vi "002_DataMonitor.vi"(11 "Queue Ref":T1={"UI"=refnum, "Message"=refnum, "Data"=refnum, "Caller"=refnum, "Name"="000 Common", "Data Path"=path "", "Class Path"=path "", "SubPanel"=refnum, "Project Name"="", "MNT"="", "Title"="", "Data Source"=refnum, "Queue List"={}, "VI"=refnum, "UE"=refnum}) -> ()   [LabVIEW 2020]
doc: "1212"
uses:
  Alin/QMH/000 Module Data Type.ctl
  Alin/QMH/Queue Message.ctl
  0007 Controls/Data Module.ctl
  0007 Controls/Data Modules.ctl
  0007 Controls/Data Element Single.ctl
  <vilib>/Utility/miscctls.llb/LVPointTypeDef.ctl
panel:
  out "QN":i32
  in  "Modules":T2={"Module01"={"Names"={"Module Name"="", "Set Value"="", "Real Value"="", "FB Value"="", "Unit"="", "Identifier"="", "IdentifierW"="写入标识符", "Decimal"="位数", "AS"=FALSE, "AR"=FALSE, "Con"=FALSE}, "Data"=[], "Digit"=0.0}, "Module02"={"Names"={"Module Name"="", "Set Value"="", "Real Value"="", "FB Value"="", "Unit"="", "Identifier"="", "IdentifierW"="写入标识符", "Decimal"="位数", "AS"=FALSE, "AR"=FALSE, "Con"=FALSE}, "Data"=[], "Digit"=0.0}, "Module03"={"Names"={"Module Name"="", "Set Value"="", "Real Value"="", "FB Value"="", "Unit"="", "Identifier"="", "IdentifierW"="写入标识符", "Decimal"="位数", "AS"=FALSE, "AR"=FALSE, "Con"=FALSE}, "Data"=[], "Digit"=0.0}, "Module04"={"Names"={"Module Name"="", "Set Value"="", "Real Value"="", "FB Value"="", "Unit"="", "Identifier"="", "IdentifierW"="写入标识符", "Decimal"="位数", "AS"=FALSE, "AR"=FALSE, "Con"=FALSE}, "Data"=[], "Digit"=0.0}, "Module05"={"Names"={"Module Name"="", "Set Value"="", "Real Value"="", "FB Value"="", "Unit"="", "Identifier"="", "IdentifierW"="写入标识符", "Decimal"="位数", "AS"=FALSE, "AR"=FALSE, "Con"=FALSE}, "Data"=[], "Digit"=0.0}, "Module06"={"Names"={"Module Name"="", "Set Value"="", "Real Value"="", "FB Value"="", "Unit"="", "Identifier"="", "IdentifierW"="写入标识符", "Decimal"="位数", "AS"=FALSE, "AR"=FALSE, "Con"=FALSE}, "Data"=[], "Digit"=0.0}, "Module07"={"Names"={"Module Name"="", "Set Value"="", "Real Value"="", "FB Value"="", "Unit"="", "Identifier"="", "IdentifierW"="写入标识符", "Decimal"="位数", "AS"=FALSE, "AR"=FALSE, "Con"=FALSE}, "Data"=[], "Digit"=0.0}, "Module08"={"Names"={"Module Name"="", "Set Value"="", "Real Value"="", "FB Value"="", "Unit"="", "Identifier"="", "IdentifierW"="写入标识符", "Decimal"="位数", "AS"=FALSE, "AR"=FALSE, "Con"=FALSE}, "Data"=[], "Digit"=0.0}, "Module09"={"Names"={"Module Name"="", "Set Value"="", "Real Value"="", "FB Value"="", "Unit"="", "Identifier"="", "IdentifierW"="写入标识符", "Decimal"="位数", "AS"=FALSE, "AR"=FALSE, "Con"=FALSE}, "Data"=[], "Digit"=0.0}, "Module10"={"Names"={"Module Name"="", "Set Value"="", "Real Value"="", "FB Value"="", "Unit"="", "Identifier"="", "IdentifierW"="写入标识符", "Decimal"="位数", "AS"=FALSE, "AR"=FALSE, "Con"=FALSE}, "Data"=[], "Digit"=0.0}, "Module11"={"Names"={"Module Name"="", "Set Value"="", "Real Value"="", "FB Value"="", "Unit"="", "Identifier"="", "IdentifierW"="写入标识符", "Decimal"="位数", "AS"=FALSE, "AR"=FALSE, "Con"=FALSE}, "Data"=[], "Digit"=0.0}}
  in  "Module Add":bool
  in  "Panel Show":bool
  in  "Panel Refresh":bool
  in  "Show Config":bool
  out "Warning":string
  in  "Horizontal scroll bar":bool caption="H"
  in  "Vertical scroll bar":bool caption="V"
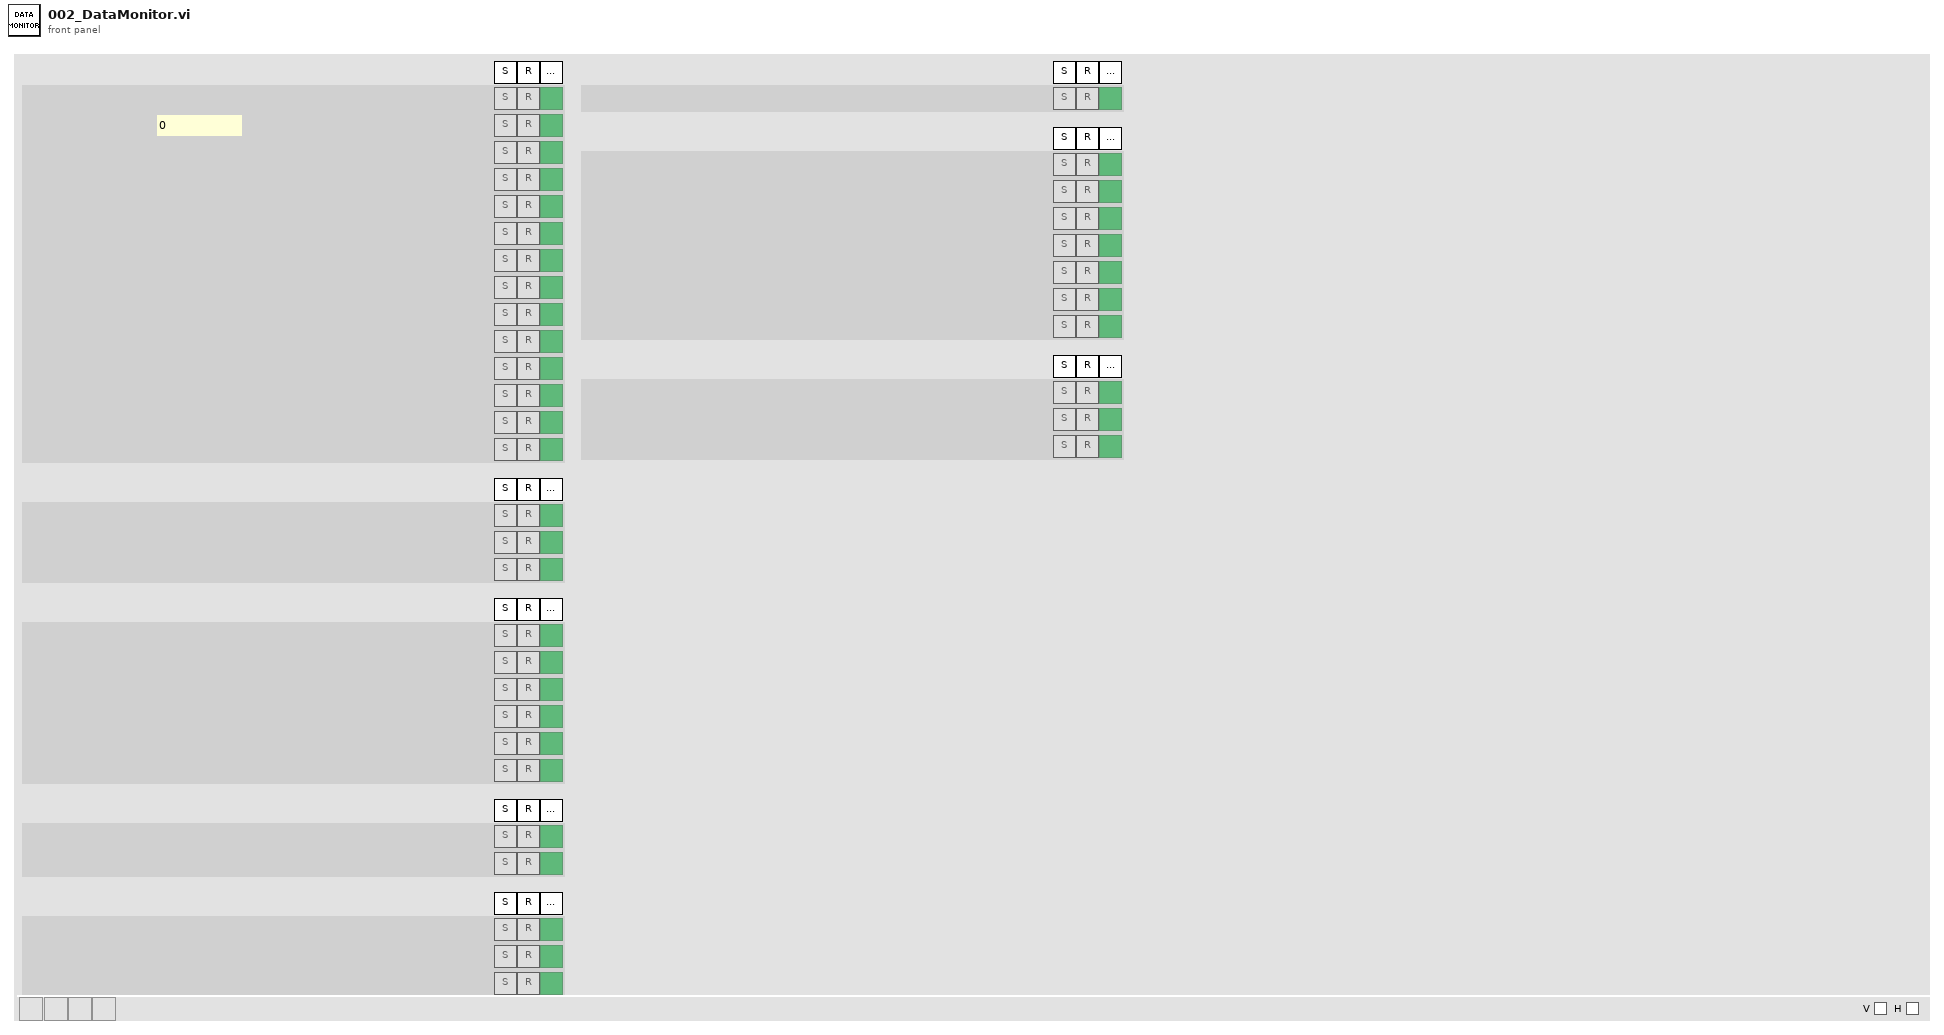
[diagram p1: front panel]
types:
  T1 = typedef "000 Module Data Type.ctl" = cluster{"UI":refnum<queue>, "Message":refnum<queue>, "Data":refnum<queue>, "Caller":refnum<queue>, "Name":string, "Data Path":path, "Class Path":path, "SubPanel":refnum<vi>, "Project Name":string, "MNT":string, "Title":string, "Data Source":refnum<queue>, "Queue List":map{string, refnum<queue>}, "VI":refnum<vi>, "UE":refnum<user-event>}
  T2 = typedef "Data Module.ctl" = cluster{"Module01":T3, "Module02":T3, "Module03":T3, "Module04":T3, "Module05":T3, "Module06":T3, "Module07":T3, "Module08":T3, "Module09":T3, "Module10":T3, "Module11":T3}
  T3 = typedef "Data Modules.ctl" = cluster{"Names":cluster{"Module Name":string, "Set Value":string, "Real Value":string, "FB Value":string, "Unit":string, "Identifier":string, "IdentifierW":string, "Decimal":string, "AS":bool, "AR":bool, "Con":bool}, "Data":T4[], "Digit":dbl}
  T4 = typedef "Data Element Single.ctl" = cluster{"Name":string, "Set Value":string, "Real Value":string, "FB Value":string, "Unit":string, "Identifier":string, "Write Name":string, "Decimal":u16, "AS":bool, "AR":bool, "ALM":bool, "Up":bool, "Down":bool}
  T5 = cluster{"Queue Ref":T1, "Modules":T2, "Count Time(ms)":u32, "Delay Time(ms)":u32, "Next":string, "WarningID":string[]}
  T6 = cluster{"Modules[0]":T3, "Modules[1]":T3, "Modules[2]":T3, "Modules[3]":T3, "Modules[4]":T3, "Modules[5]":T3, "Modules[6]":T3, "Modules[7]":T3, "Modules[8]":T3, "Modules[9]":T3, "Modules[10]":T3}
  T7 = typedef "SDQ Data Type.ctl" = cluster{"CAN Length":string, "CAN Name":string, "CAN ID":string, "CAN Type":string, "Test Item":string, "Byte Order":string, "Instruction":string, "Control Type":string, "Group":string, "Offset":dbl, "Coefficient":dbl, "Write Enable":bool, "Lable Type":string, "Key?":string, "Set Value":string, "Upper":dbl, "Lower":dbl, "Unit":string, "Formula":string, "Test Item Type":string, "Length":i32, "Address":string, "Name":string, "Identifier":string, "Data Type":string, "Enumerate?":string, "Enumerate List":string, "Data":string, "Source":string}
  T8 = cluster{"[0]":T3, "[1]":T3, "[2]":T3, "[3]":T3, "[4]":T3, "[5]":T3, "[6]":T3, "[7]":T3, "[8]":T3, "[9]":T3, "[10]":T3}
  T9 = typedef "eventvkey.ctl" = enum16{"ASCII", "Enter", "Return", "Shift", "Ctrl", "Alt", "Cmd", "Opt", "Caps", "NumLock", "Clear", "Break", "Up", "Down", "Left", "Right", "Insert", "Delete", "Home", "End", "PageUp", "PageDown", "Escape", "Help", "Pause", "ScrollLock", "F1", "F2", "F3", "F4", "F5", "F6", "F7", "F8", "F9", "F10", "F11", "F12", "F13", "F14", "F15", "F16", "F17", "F18", "F19", "F20", "F21", "F22", "F23", "F24", "Play", "VolumeUp", "VolumeDown", "Mute", "Two Byte Char"}
  T10 = cluster{"Shift":bool, "Ctrl":bool, "Alt":bool, "Cmd":bool, "Opt":bool}
  T11 = typedef "LVPoint32TypeDef.ctl" = cluster{"Horizontal":i32, "Vertical":i32}
  T12 = cluster{"Queue List":map{string, refnum<queue>}, "SubPanel":refnum<vi>, "Active Panel":string, "Queue Ref":T1, "Project Name":string, "ModulesRef":refnum<vi>, "Vertical scroll bar":bool, "Horizontal scroll bar":bool}
  T13 = typedef "LVPointTypeDef.ctl" = cluster{"Horizontal":i16, "Vertical":i16}
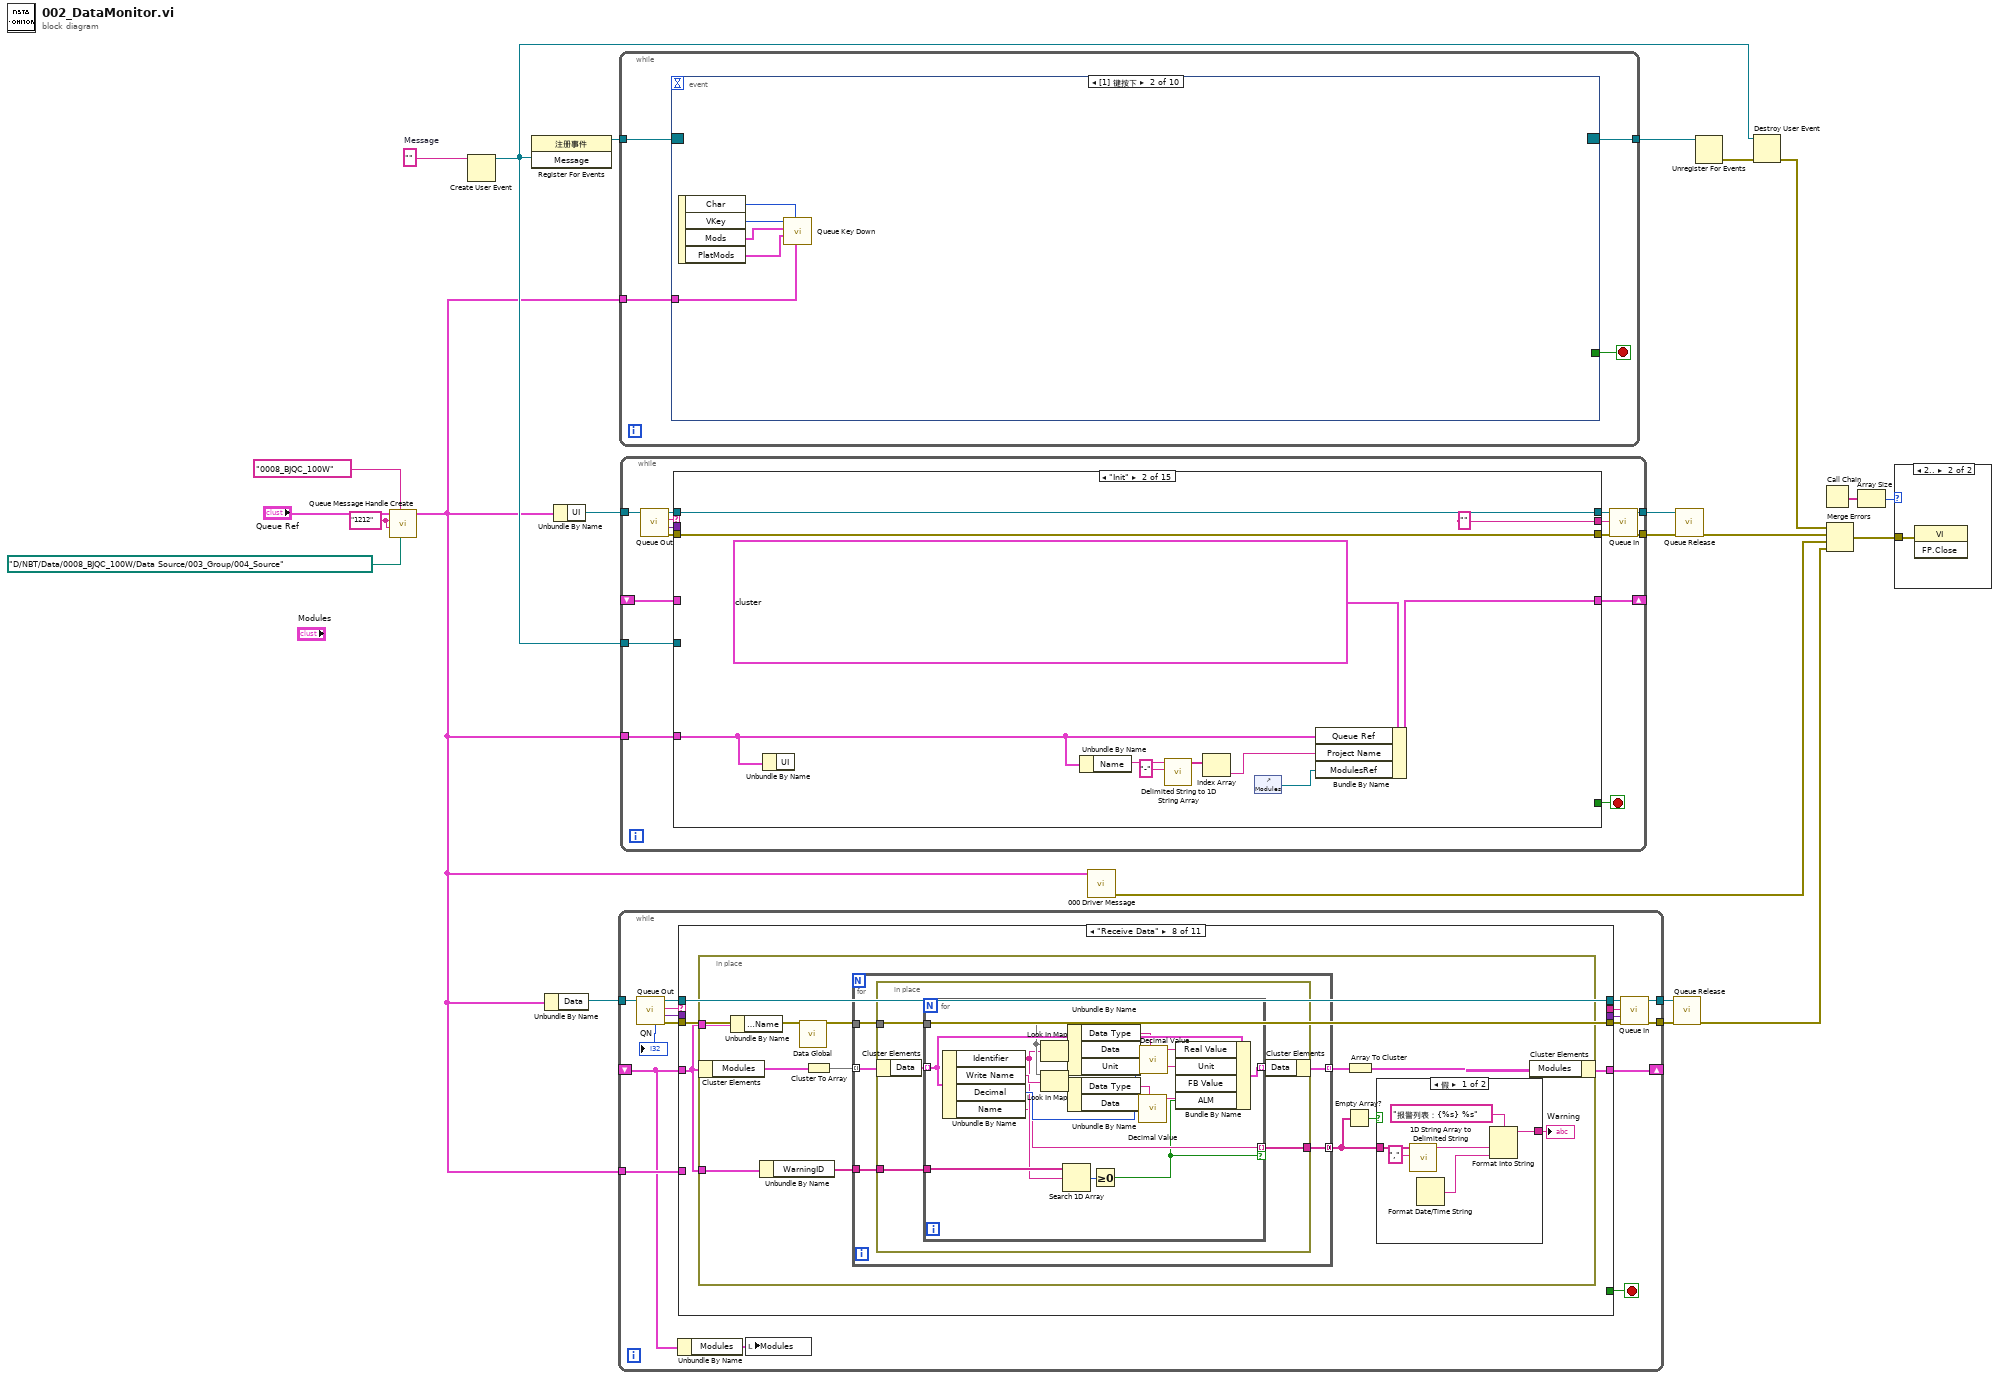
[diagram p0: block diagram]
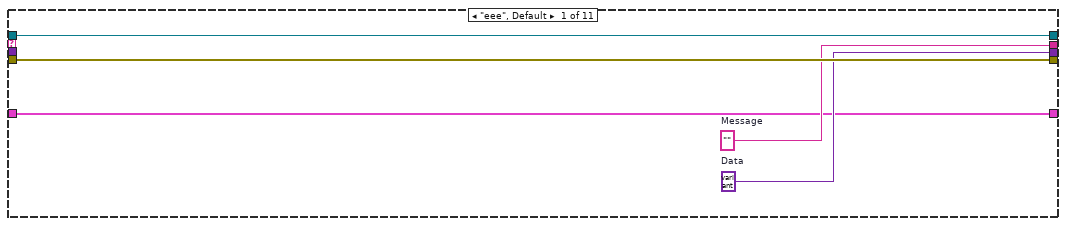
[diagram p2: hidden frame]
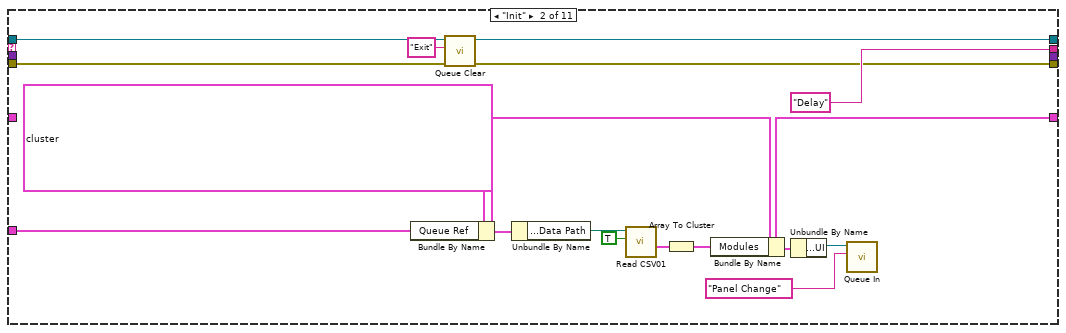
[diagram p3: hidden frame]
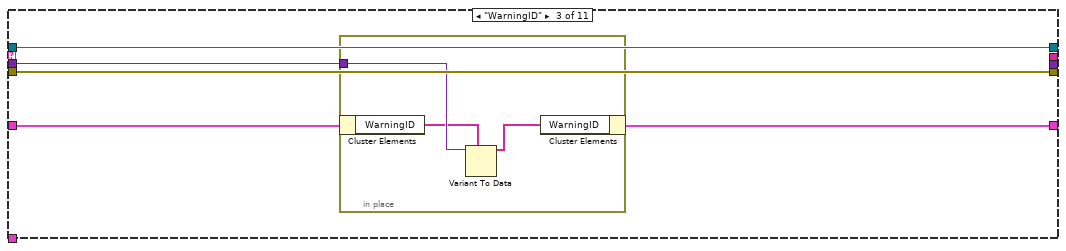
[diagram p4: hidden frame]
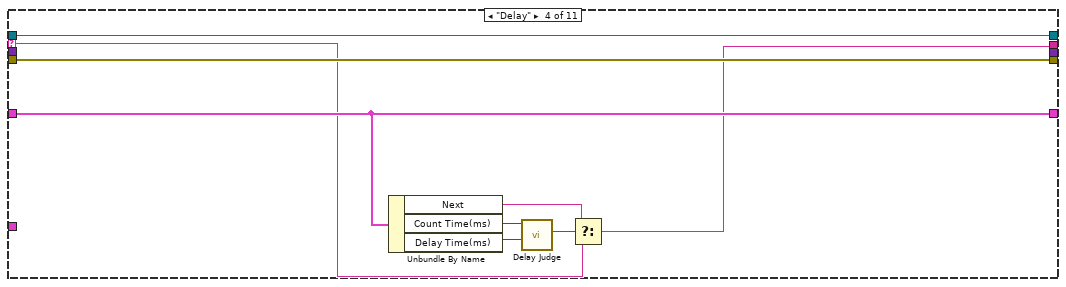
[diagram p5: hidden frame]
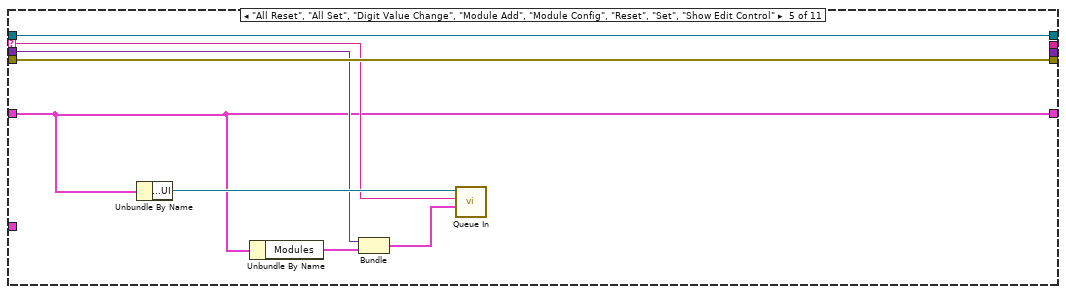
[diagram p6: hidden frame]
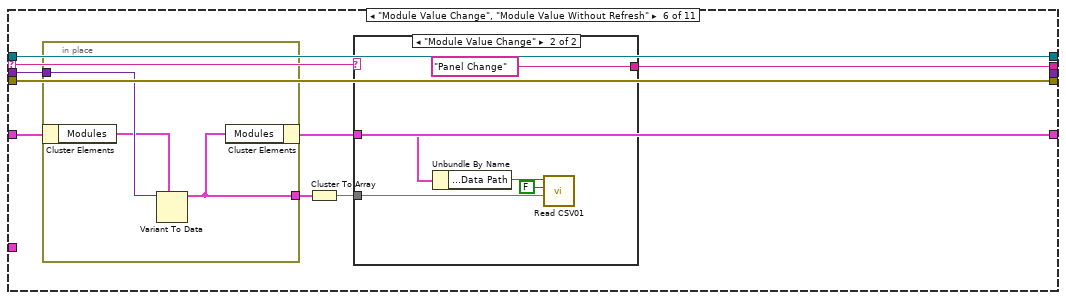
[diagram p7: hidden frame]
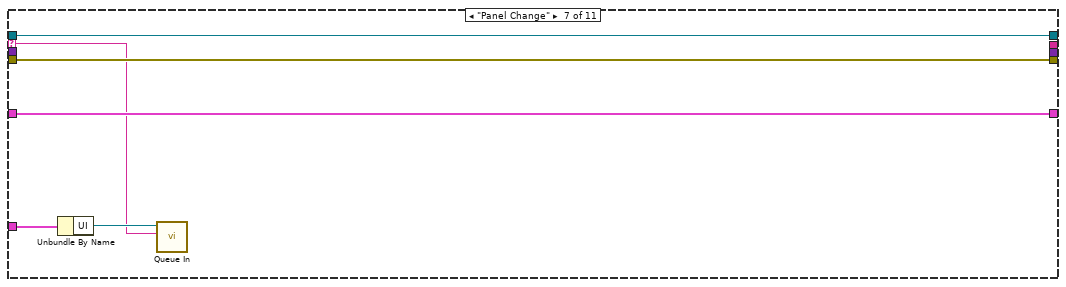
[diagram p9: hidden frame]
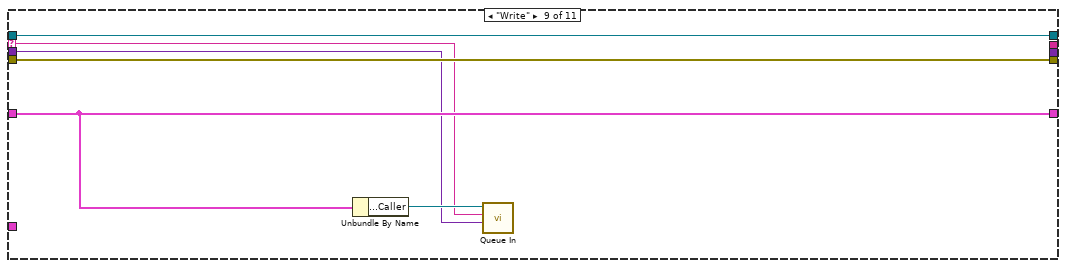
[diagram p11: hidden frame]
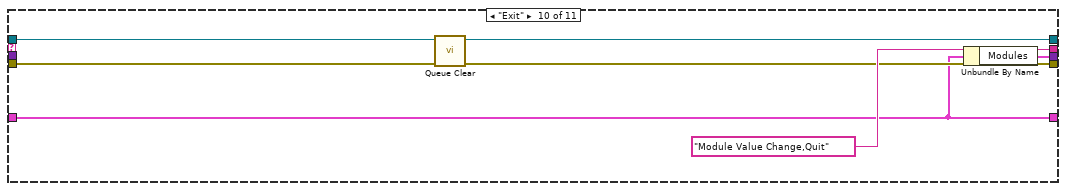
[diagram p12: hidden frame]
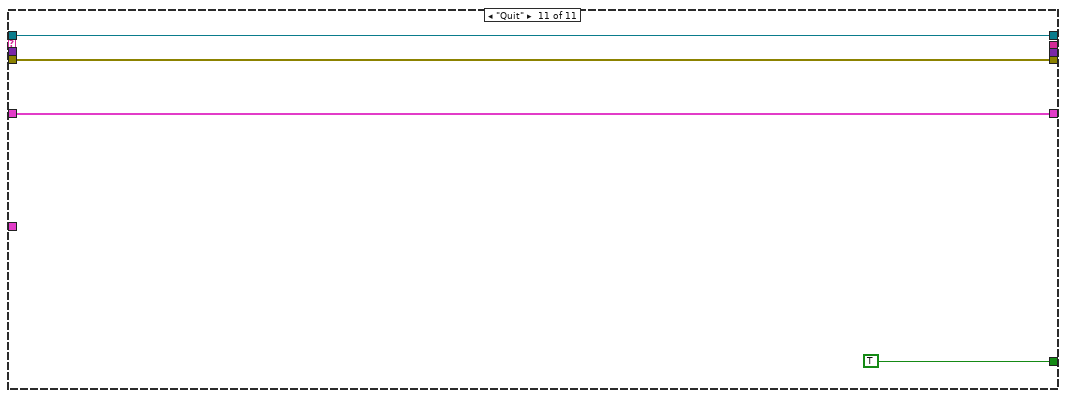
[diagram p13: hidden frame]
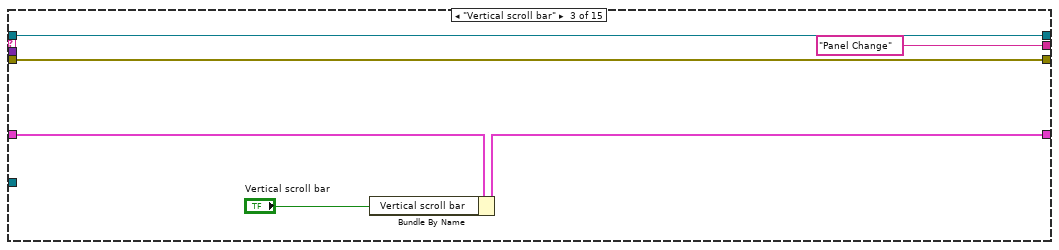
[diagram p16: hidden frame]
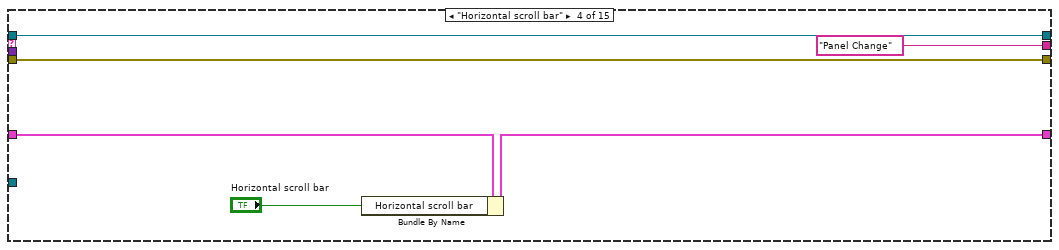
[diagram p17: hidden frame]
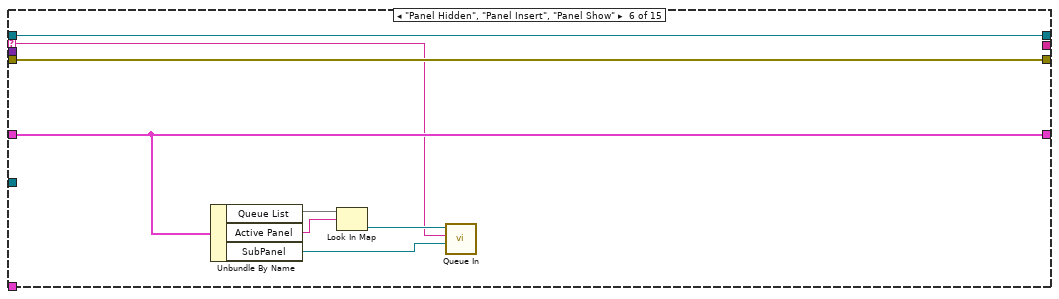
[diagram p19: hidden frame]
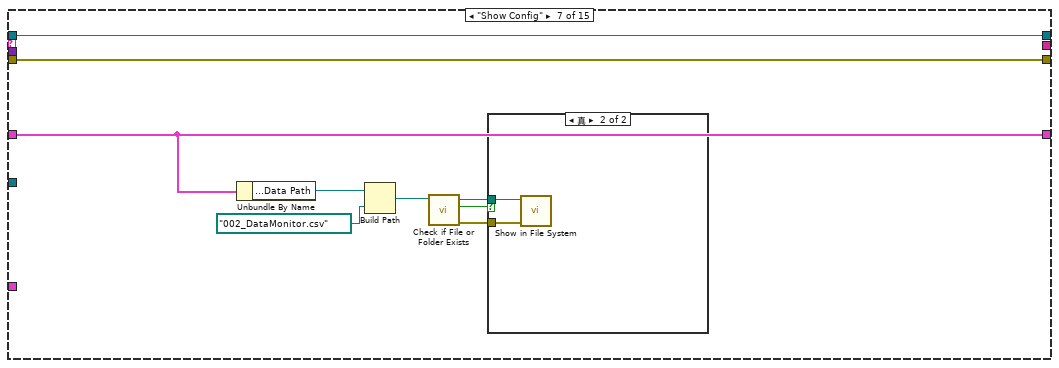
[diagram p20: hidden frame]
diagram:
  w1 = "1212" ("Title")
  w6 = ""  # Message
  n1 = call "Queue Message Handle Create.vi"("Data Path"=path "D:/NBT/Data/0008_BJQC_100W/Data Source/003_Group/004_Source", "Project Name"="0008_BJQC_100W", "Name"=w1, "Title"=w1, "Queue Ref In"="Queue Ref") -> ("Queue Ref Out"=w5:T1)  [unwired: 5 in, 1 out]
  n2 = Create User Event(user event datatype=w6) -> (user event=w10:refnum<user-event>)  [unwired: 1 in, 1 out]
  n3 = register-events(w10) -> (reference out=w7:refnum<event-registration>)  [unwired: 2 in, 1 out]
  n4 = Unbundle By Name(w5) -> ("Data"=w21:refnum<queue>)
  n5 = Unbundle By Name(w5) -> ("UI"=w13:refnum<queue>)
  n6 = while {
    tunnel: w21 -> [w36]
    tunnel: [w33] -> w19
    tunnel: [w32] -> w20
    shift-right: [w25] -> _
    shift-left: _ -> [w24]
    tunnel: w5 -> [w28]
    stop <- w40 stop-if-true
    n7 = call "Queue Out.vi"("Queue In"=w36) -> ("error out"=w39:errorcluster, "Data"=w37:variant, "Message"=w38:string, "Queue Out"=w35:refnum<queue>, "Queue NUmber"=→"QN":i32)  [unwired: 6 in]
    n8 = Unbundle By Name(w24) -> ("Modules"=w26:T2)
    n9 = case shown="\"Receive Data\"" w38 {
      selector: w38 -> [_ _ _ w71 w83 w89 w104 _ w162 _ _]
      tunnel: w35 -> [w45 w48 w66 w78 w86 w95 w109 w113 w166 w172 w176]
      tunnel: w39 -> [w44 w61 w65 w77 w85 w94 w108 w112 w165 w170 w177]
      tunnel: [w45 w47 w66 w78 w86 w95 w109 w113 w166 w171 w176] -> w34
      tunnel: [w44 w49 w65 w77 w85 w94 w108 w112 w165 w169 w177] -> w31
      tunnel: [w43 "Delay" ("Message") _ w70 _ w91 _ _ _ "Module Value Change,Quit" _] -> w30
      tunnel: [_ _ _ _ _ _ _ _ _ _ TRUE] -> w40
      tunnel: [w42 _ _ _ _ _ _ _ _ w167 _] -> w29
      tunnel: w37 -> [_ _ w62 _ w82 w92 _ _ w161 _ _]
      tunnel: [w41 w52 w63 w76 w81 w87 w107 w111 w164 w168 w174] -> w25
      tunnel: w24 -> [w41 _ w64 w76 w81 w93 w107 w110 w164 w168 w174]
      tunnel: w28 -> [_ w59 _ _ _ _ w106 _ _ _ _]
      frame "eee", Default {
        w42 = variant  # Data
        w43 = ""  # Message
      }
      frame "Init" {
        n10 = Bundle By Name(cluster=T5 {"Queue Ref"={"UI"=refnum, "Message"=refnum, "Data"=refnum, "Caller"=refnum, "Name"="", "Data Path"=path "", "Class Path"=path "", "SubPanel"=refnum, "Project Name"="", "MNT"="", "Title"="", "Data Source"=refnum, "Queue List"={}, "VI"=refnum, "UE"=refnum}, "Modules"={"Module01"={"Names"={"Module Name"="", "Set Value"="", "Real Value"="", "FB Value"="", "Unit"="", "Identifier"="", "IdentifierW"="写入标识符", "Decimal"="位数", "AS"=FALSE, "AR"=FALSE, "Con"=FALSE}, "Data"=[], "Digit"=0.0}, "Module02"={"Names"={"Module Name"="", "Set Value"="", "Real Value"="", "FB Value"="", "Unit"="", "Identifier"="", "IdentifierW"="写入标识符", "Decimal"="位数", "AS"=FALSE, "AR"=FALSE, "Con"=FALSE}, "Data"=[], "Digit"=0.0}, "Module03"={"Names"={"Module Name"="", "Set Value"="", "Real Value"="", "FB Value"="", "Unit"="", "Identifier"="", "IdentifierW"="写入标识符", "Decimal"="位数", "AS"=FALSE, "AR"=FALSE, "Con"=FALSE}, "Data"=[], "Digit"=0.0}, "Module04"={"Names"={"Module Name"="", "Set Value"="", "Real Value"="", "FB Value"="", "Unit"="", "Identifier"="", "IdentifierW"="写入标识符", "Decimal"="位数", "AS"=FALSE, "AR"=FALSE, "Con"=FALSE}, "Data"=[], "Digit"=0.0}, "Module05"={"Names"={"Module Name"="", "Set Value"="", "Real Value"="", "FB Value"="", "Unit"="", "Identifier"="", "IdentifierW"="写入标识符", "Decimal"="位数", "AS"=FALSE, "AR"=FALSE, "Con"=FALSE}, "Data"=[], "Digit"=0.0}, "Module06"={"Names"={"Module Name"="", "Set Value"="", "Real Value"="", "FB Value"="", "Unit"="", "Identifier"="", "IdentifierW"="写入标识符", "Decimal"="位数", "AS"=FALSE, "AR"=FALSE, "Con"=FALSE}, "Data"=[], "Digit"=0.0}, "Module07"={"Names"={"Module Name"="", "Set Value"="", "Real Value"="", "FB Value"="", "Unit"="", "Identifier"="", "IdentifierW"="写入标识符", "Decimal"="位数", "AS"=FALSE, "AR"=FALSE, "Con"=FALSE}, "Data"=[], "Digit"=0.0}, "Module08"={"Names"={"Module Name"="", "Set Value"="", "Real Value"="", "FB Value"="", "Unit"="", "Identifier"="", "IdentifierW"="写入标识符", "Decimal"="位数", "AS"=FALSE, "AR"=FALSE, "Con"=FALSE}, "Data"=[], "Digit"=0.0}, "Module09"={"Names"={"Module Name"="", "Set Value"="", "Real Value"="", "FB Value"="", "Unit"="", "Identifier"="", "IdentifierW"="写入标识符", "Decimal"="位数", "AS"=FALSE, "AR"=FALSE, "Con"=FALSE}, "Data"=[], "Digit"=0.0}, "Module10"={"Names"={"Module Name"="", "Set Value"="", "Real Value"="", "FB Value"="", "Unit"="", "Identifier"="", "IdentifierW"="写入标识符", "Decimal"="位数", "AS"=FALSE, "AR"=FALSE, "Con"=FALSE}, "Data"=[], "Digit"=0.0}, "Module11"={"Names"={"Module Name"="", "Set Value"="", "Real Value"="", "FB Value"="", "Unit"="", "Identifier"="", "IdentifierW"="写入标识符", "Decimal"="位数", "AS"=FALSE, "AR"=FALSE, "Con"=FALSE}, "Data"=[], "Digit"=0.0}}, "Count Time(ms)"=150, "Delay Time(ms)"=150, "Next"="Receive Data,Delay", "WarningID"=[]}, "Queue Ref"=w59) -> (w58:T5)
        n11 = call "Queue Clear.vi"("error in (no error)"=w61, "Filter"="Exit", "Queue In"=w48) -> ("error out"=w49:errorcluster, "Queue Out"=w47:refnum<queue>)  [unwired: 7 in]
        n12 = Unbundle By Name(w58) -> ("Queue Ref.Data Path"=w56:path)
        n13 = call "Read CSV01.vi"("Read?"=TRUE, "Data Monitor"=w56) -> ("Modules"=w54:T3[])  [unwired: 8 in, 1 out]
        n14 = Array To Cluster(array=w54) -> (cluster=w57:T6)
        n15 = Bundle By Name(cluster=w58, "Modules"=w57) -> (w52:T5)
        n16 = Unbundle By Name(w52) -> ("Queue Ref.UI"=w51:refnum<queue>)
        n17 = call "Queue In.vi"("Message"="Panel Change", "Queue In"=w51) -> ()  [unwired: 8 in, 2 out]
      }
      frame "WarningID" {
        n18 = in-place {
          in-place-border: w62 -> [w69]
          n19 = in-place-cluster #1(w64) -> ("WarningID"=w68:string[])
          n20 = Variant To Data(type=w68, Variant=w69) -> (data=w67:string[])  [unwired: 1 in, 1 out]
          n21 = in-place-cluster #1("WarningID"=w67) -> (w63:T5)
        }
      }
      frame "Delay" {
        n22 = Unbundle By Name(w76) -> ("Next"=w72:string, "Count Time(ms)"=w75:u32, "Delay Time(ms)"=w74:u32)
        n23 = call "Delay Judge.vi"("Delay Time(ms)"=w74, "Count Time(ms)"=w75) -> ("Time Out?"=w73:bool)  [unwired: 5 in, 4 out]
        n24 = Select(t=w72, s=w73, f=w71) -> (s? t:f=w70:string)
      }
      frame "All Reset", "All Set", "Digit Value Change", "Module Add", "Module Config", "Reset", "Set", "Show Edit Control" {
        n25 = Unbundle By Name(w81) -> ("Queue Ref.UI"=w84:refnum<queue>)
        n26 = Unbundle By Name(w81) -> ("Modules"=w79:T2)
        n27 = Bundle("Data"=w82, "Modules"=w79) -> (w80:cluster{"Data":variant, "Modules":T2})  [unwired: 1 in]
        n28 = call "Queue In.vi"("Data"=w80, "Message"=w83, "Queue In"=w84) -> ()  [unwired: 7 in, 2 out]
      }
      frame "Module Value Change", "Module Value Without Refresh" {
        n29 = in-place {
          in-place-border: w92 -> [w103]
          in-place-border: [w101] -> w90
          n30 = in-place-cluster #2(w93) -> ("Modules"=w102:T2)
          n31 = Variant To Data(type=w102, Variant=w103) -> (data=w101:T2)  [unwired: 1 in, 1 out]
          n32 = in-place-cluster #2("Modules"=w101) -> (w87:T5)
        }
        n33 = Cluster To Array(cluster=w90) -> (array=w88:T3[])
        n34 = case shown="\"Module Value Change\"" w89 {
          tunnel: [_ "Panel Change" ("Message")] -> w91
          tunnel: w88 -> [_ w99]
          tunnel: w87 -> [_ w98]
          frame "eee", Default {
          }
          frame "Module Value Change" {
            n35 = Unbundle By Name(w98) -> ("Queue Ref.Data Path"=w97:path)
            n36 = call "Read CSV01.vi"("Modules In"=w99, "Read?"=FALSE, "Data Monitor"=w97) -> ()  [unwired: 7 in, 2 out]
          }
        }
      }
      frame "Panel Change" {
        n37 = Unbundle By Name(w106) -> ("UI"=w105:refnum<queue>)
        n38 = call "Queue In.vi"("Message"=w104, "Queue In"=w105) -> ()  [unwired: 8 in, 2 out]
      }
      frame "Receive Data" {
        n39 = in-place {
          in-place-border: w110 -> [w120]
          in-place-border: w110 -> [w118]
          n40 = in-place-cluster #3(w110) -> ("Modules"=w123:T2)
          n41 = Unbundle By Name(w120) -> ("Queue Ref.Name"=w119:string)
          n42 = Unbundle By Name(w118) -> ("WarningID"=w117:string[])
          n43 = call "Data Global.vi"("Name"=w119) -> ("Data Out"=w121:map{string, T7})  [unwired: 7 in, 3 out]
          n44 = Cluster To Array(cluster=w123) -> (array=w124:T3[])
          n45 = for {
            tunnel: w124 -> [w136] mode=indexing
            tunnel: [w135] -> w125 mode=indexing
            tunnel: w121 -> [w134]
            tunnel: w117 -> [w133]
            tunnel: [w132] -> w115 mode=concatenating
            n46 = in-place {
              in-place-border: w134 -> [w140]
              in-place-border: w133 -> [w138]
              in-place-border: [w137] -> w132
              n47 = in-place-cluster #4(w136) -> ("Data"=w141:T4[])
              n48 = for {
                tunnel: w141 -> [w160] mode=indexing
                tunnel: w140 -> [w159]
                tunnel: [w157] -> w139 mode=indexing
                tunnel: w138 -> [w148]
                tunnel: [w145] -> w137 mode=indexing if=w144
                n49 = Unbundle By Name(w160) -> ("Identifier"=w147:string, "Write Name"=w155:string, "Decimal"=w150:u16, "Name"=w145:string)
                n50 = Look In Map(map=w159, key=w147) -> (value=w158:T7)  [unwired: 1 in, 1 out]
                n51 = Look In Map(map=w159, key=w155) -> (value=w156:T7)  [unwired: 1 in, 1 out]
                n52 = Search 1D Array(1D array=w148, element=w147) -> (index of element=w146:i32)  [unwired: 1 in]
                n53 = Unbundle By Name(w158) -> ("Data Type"=w143:string, "Data"=w149:string, "Unit"=w154:string)
                n54 = Unbundle By Name(w156) -> ("Data Type"=w142:string, "Data"=w153:string)
                n55 = Greater Or Equal To 0?(x=w146) -> (x >= 0?=w144:bool)
                n56 = call "Decimal Value.vi"("Type"=w142, "Decimal"=w150, "Data In"=w153) -> ("Data Out"=w152:string)  [unwired: 8 in]
                n57 = call "Decimal Value.vi"("Type"=w143, "Decimal"=w150, "Data In"=w149) -> ("Data Out"=w151:string)  [unwired: 8 in]
                n58 = Bundle By Name(cluster=w160, "Real Value"=w151, "Unit"=w154, "FB Value"=w152, "ALM"=w144) -> (w157:T4)
              }
              n59 = in-place-cluster #4("Data"=w139) -> (w135:T3)
            }
          }
          n60 = Empty Array?(array=w115) -> (empty?=w114:bool)
          n61 = Array To Cluster(array=w125) -> (cluster=w122:T8)
          n62 = case shown="假" w114 {
            tunnel: [w126 _] -> w116
            tunnel: w115 -> [w130 _]
            frame False {
              n63 = call <vilib>:"1D String Array to Delimited String.vi"("delimiter"=",", "string array"=w130) -> ("delimited string"=w127:string)  [unwired: 9 in]
              n64 = Format Date/Time String() -> (date/time string=w129:string)  [unwired: 3 in]
              n65 = Format Into String(format string="报警列表：{%s} %s" ("格式字符串"), w127, w129) -> (resulting string=w126:string)  [unwired: 2 in, 1 out]
            }
            frame True {
            }
          }
          "Warning" <- w116
          n66 = in-place-cluster #3("Modules"=w122) -> (w111:T5)
        }
      }
      frame "Write" {
        n67 = Unbundle By Name(w164) -> ("Queue Ref.Caller"=w163:refnum<queue>)
        n68 = call "Queue In.vi"("Data"=w161, "Message"=w162, "Queue In"=w163) -> ()  [unwired: 7 in, 2 out]
      }
      frame "Exit" {
        n69 = call "Queue Clear.vi"("error in (no error)"=w170, "Queue In"=w172) -> ("error out"=w169:errorcluster, "Queue Out"=w171:refnum<queue>)  [unwired: 8 in]
        n70 = Unbundle By Name(w168) -> ("Modules"=w167:T2)
      }
      frame "Quit" {
      }
    }
    n71 = local write "Modules"(w26) -> ()
    n72 = call "Queue In.vi"("error in (no error)"=w31, "Data"=w29, "Message"=w30, "Queue In"=w34) -> ("error out"=w32:errorcluster, "Queue Out"=w33:refnum<queue>)  [unwired: 6 in]
  }
  n73 = while {
    tunnel: w7 -> [w181]
    tunnel: [w179] -> w8
    tunnel: w5 -> [w178]
    stop <- w180 stop-if-true
    n74 = event shown="[1] 键按下" {
      selector: w181 -> [_ _ _ _ _ _ _ _ _ _]
      dyn-events: [_ _ _ _ _ _ _ _ _ _] -> w179
      timeout: _ -> [_ _ _ _ _ _ _ _ _ _]
      tunnel: [_ _ _ w190 _ _ _ _ _ _] -> w180
      tunnel: w178 -> [_ w185 w189 _ w197 w206 w217 w250 w259 w263]
      event Timeout {
        n75 = event-data() -> ()  [unwired: 1 in, 1 out]
      }
      event Key Down {
        n76 = event-data() -> ("Char"=w186:i16, "VKey"=w184:T9, "Mods"=w183:cluster{"Num Pad":bool, "Menu Key":bool}, "PlatMods"=w182:T10)  [unwired: 1 in]
        n77 = call "Queue Key Down.vi"("Queue Ref Out"=w185, "C"=w186, "Platform Key"=w182, "Group Key"=w183, "V Key"=w184) -> ()  [unwired: 6 in, 1 out]
      }
      event Panel Resize {
        n78 = event-data() -> ()  [unwired: 1 in, 1 out]
        n79 = Unbundle By Name(w189) -> ("Message"=w188:refnum<queue>)
        n80 = call "Queue In.vi"("Message"="Panel Change", "Queue In"=w188) -> ()  [unwired: 8 in, 2 out]
      }
      event User Event {
        n81 = event-data() -> ("Message"=w192:string)  [unwired: 1 in]
        n82 = Equal?(x=w192, y="Exit") -> (x = y?=w190:bool)
      }
      event Mouse Down {
        n83 = event-data() -> ("CtlRef"=w199:refnum<vi>, "Coords"=w198:T11)  [unwired: 1 in, 3 out]
        n84 = Unbundle By Name(w197) -> ("Data"=w196:refnum<queue>)
        n85 = call "Move Position.vi"("Position"=w198, "Array Ref"=w199) -> ("OK?"=w193:bool, "Index"=w195:cluster{i32, u32, "Value":dbl})  [unwired: 7 in, 1 out]
        n86 = case shown="真" w193 {
          tunnel: w196 -> [_ w202]
          tunnel: w195 -> [_ w201]
          tunnel: "Show Edit Control" ("Message") -> [_ w200]
          frame False {
          }
          frame True {
            n87 = call "Queue In.vi"("Data"=w201, "Message"=w200, "Queue In"=w202) -> ()  [unwired: 7 in, 2 out]
          }
        }
      }
      event "Module Add": Value Change {
        n88 = event-data() -> ("CtlRef"=w207:refnum<vi>)  [unwired: 1 in]
        n89 = Unbundle By Name(w206) -> ("Data"=w205:refnum<queue>)
        n90 = property class="Bool"(reference=w207) -> ("Label.Text"=w204:string)  [unwired: 1 in, 2 out]
        n91 = call "Queue In.vi"("Data"=cluster{i32, i32, "Digit":dbl} {0, 0, "Digit"=0.0} ("输出簇"), "Message"=w204, "Queue In"=w205) -> ()  [unwired: 7 in, 2 out]
      }
      event Value Change {
        n92 = event-data() -> ("OldVal"=w210:T2, "NewVal"=w209:T2)  [unwired: 1 in]
        n93 = Unbundle By Name(w217) -> ("Data"=w208:refnum<queue>)
        n94 = Cluster To Array(cluster=w210) -> (array=w214:T3[])
        n95 = Cluster To Array(cluster=w209) -> (array=w212:T3[])
        n96 = for {
          tunnel: w212 -> [w241] mode=indexing
          tunnel: [w229] -> w213
          tunnel: w214 -> [w233] mode=indexing
          tunnel: "All Set\nAll Reset\nModule Config\nSet\nReset\nDigit Value Change\nDrop Value Change" ("Message") -> [w231]
          tunnel: [w228] -> w215
          tunnel: [w224] -> w216
          i -> [w226]
          stop <- w234 stop-if-true
          n97 = Unbundle By Name(w241) -> ("Digit"=w221:dbl, "Names.AS"=w232:bool, "Names.AR"=w239:bool, "Names.Con"=w238:bool, "Data"=w240:T4[])
          n98 = Unbundle By Name(w233) -> ("Digit"=w222:dbl)
          n99 = Not Equal?(x=w222, y=w221) -> (x != y?=w223:bool)
          n100 = for {
            tunnel: w240 -> [w248] mode=indexing
            tunnel: [w246] -> w237
            tunnel: [w245] -> w236
            tunnel: [w244] -> w225
            i -> [w244]
            stop <- w247 stop-if-true
            n101 = Unbundle By Name(w248) -> ("AS"=w246:bool, "AR"=w245:bool)
            n102 = Compound Arithmetic op=OR ("复合运算")(w246, w245) -> (w247:bool)
          }
          n103 = Build Array(w232, w239, w238, w237, w236, w223) -> (w235:bool[])
          n104 = Bundle(w226, w225, "Digit"=w221) -> (w227:cluster{i32, i32, "Digit":dbl})  [unwired: 1 in]
          n105 = Or Array Elements(Boolean array=w235) -> (logical OR=w234:bool)
          n106 = To Variant(anything=w227) -> (Variant=w224:variant)
          n107 = for {
            tunnel: w235 -> [w242] mode=indexing
            tunnel: [w243] -> w230
            tunnel: [w242] -> w229
            i -> [w243]
            stop <- w242 stop-if-true
          }
          n108 = Pick Line(multi-line string=w231, line index=w230) -> (output string=w228:string)  [unwired: 1 in]
        }
        n109 = case shown="真" w213 {
          tunnel: w215 -> [_ w218]
          tunnel: w216 -> [_ w220]
          tunnel: w208 -> [_ w219]
          frame False {
          }
          frame True {
            n110 = call "Queue In.vi"("Data"=w220, "Message"=w218, "Queue In"=w219) -> ()  [unwired: 7 in, 2 out]
          }
        }
      }
      event Panel Close? {
        n111 = event-data() -> ()  [unwired: 1 in, 1 out]
        n112 = Unbundle By Name(w250) -> ("Message"=w249:refnum<queue>)
        n113 = Call Chain() -> (call chain=w253:string[])
        n114 = Array Size(array=w253) -> (size(s)=w252:i32)
        n115 = case shown="0, 默认" w252 {
          tunnel: ["Exit Prepare" ("Message") "Panel Hidden" ("Message")] -> w251
          frame 0, Default {
          }
          frame 2.. {
          }
        }
        n116 = call "Queue In.vi"("Message"=w251, "Queue In"=w249) -> ()  [unwired: 8 in, 2 out]
        n117 = event-data("Discard?"=TRUE ("放弃？")) -> ()  [unwired: 1 in, 1 out]
      }
      event "Show Config", "Panel Refresh", "Vertical scroll bar", "Horizontal scroll bar": Value Change {
        n118 = event-data() -> ("CtlRef"=w260:refnum<vi>)  [unwired: 1 in]
        n119 = property class="Bool"(reference=w260) -> ("Label.Text"=w257:string)  [unwired: 1 in, 2 out]
        n120 = Unbundle By Name(w259) -> ("UI"=w258:refnum<queue>)
        n121 = call "Queue In.vi"("Message"=w257, "Queue In"=w258) -> ()  [unwired: 8 in, 2 out]
      }
      event "Panel Show": Value Change {
        n122 = event-data() -> ("CtlRef"=w264:refnum<vi>)  [unwired: 1 in]
        n123 = Unbundle By Name(w263) -> ("Message"=w262:refnum<queue>)
        n124 = property class="Bool"(reference=w264) -> ("Label.Text"=w261:string)  [unwired: 1 in, 2 out]
        n125 = call "Queue In.vi"("Message"=w261, "Queue In"=w262) -> ()  [unwired: 8 in, 2 out]
      }
    }
  }
  n126 = while {
    tunnel: w13 -> [w274]
    tunnel: [w271] -> w11
    tunnel: [w270] -> w12
    tunnel: w10 -> [w278]
    tunnel: w5 -> [w267]
    shift-right: [w266] -> _
    shift-left: _ -> [w265]
    stop <- w279 stop-if-true
    n127 = call "Queue Out.vi"("Queue In"=w274) -> ("error out"=w277:errorcluster, "Data"=w275:variant, "Message"=w276:string, "Queue Out"=w273:refnum<queue>)  [unwired: 6 in, 1 out]
    n128 = case shown="\"Init\"" w276 {
      selector: w276 -> [_ _ _ _ _ w311 _ _ w339 w346 w360 _ w372 w376 _]
      tunnel: w273 -> [w282 w293 w299 w305 w308 w316 w325 w332 w340 w354 w364 w367 w374 w384 w392]
      tunnel: w277 -> [w281 w292 w298 w304 w307 w315 w324 w331 w338 w353 w363 w366 w373 w382 w393]
      tunnel: [w282 w293 w299 w305 w308 w316 w325 w332 w341 w354 w364 w367 w374 w383 w392] -> w272
      tunnel: [w281 w292 w298 w304 w307 w315 w324 w331 w342 w353 w363 w366 w373 w381 w393] -> w269
      tunnel: [_ "" "Panel Change" "Panel Change" _ _ _ _ _ _ _ _ _ "Quit" _] -> w268
      tunnel: [_ _ _ _ _ _ _ _ _ _ _ _ _ _ TRUE] -> w279
      tunnel: w278 -> [_ _ _ _ _ _ _ _ _ _ _ _ _ w386 _]
      tunnel: w275 -> [_ _ _ _ _ _ _ _ _ w350 _ _ w368 _ _]
      tunnel: w267 -> [_ w283 _ _ _ _ _ _ _ w349 w362 _ w371 w380 _]
      tunnel: [w280 w290 w296 w302 w306 w314 w323 w330 w337 w351 w359 w365 w370 w375 w390] -> w266
      tunnel: w265 -> [w280 _ w297 w303 w306 w314 w323 w330 w337 w352 w359 w365 w370 w375 w390]
      frame "eee", Default {
      }
      frame "Init" {
        n129 = Unbundle By Name(w283) -> ()  [unwired: 1 out]
        n130 = Unbundle By Name(w283) -> ("Name"=w289:string)
        n131 = call <vilib>:"Delimited String to 1D String Array.vi"("delimiter"="-", "delimited string"=w289) -> ("string array"=w287:string[])  [unwired: 9 in]
        n132 = Index Array(array=w287) -> (element=w286:string)  [unwired: 1 in]
        n133 = control-ref of="Modules"() -> (w285:refnum<vi>)
        n134 = Bundle By Name(cluster=T12 {"Queue List"={}, "SubPanel"=refnum, "Active Panel"="", "Queue Ref"={"UI"=refnum, "Message"=refnum, "Data"=refnum, "Caller"=refnum, "Name"="", "Data Path"=path "", "Class Path"=path "", "SubPanel"=refnum, "Project Name"="", "MNT"="", "Title"="", "Data Source"=refnum, "Queue List"={}, "VI"=refnum, "UE"=refnum}, "Project Name"="", "ModulesRef"=refnum, "Vertical scroll bar"=FALSE, "Horizontal scroll bar"=FALSE}, "Queue Ref"=w283, "Project Name"=w286, "ModulesRef"=w285) -> (w290:T12)
      }
      frame "Vertical scroll bar" {
        n135 = Bundle By Name(cluster=w297, "Vertical scroll bar"="Vertical scroll bar") -> (w296:T12)
      }
      frame "Horizontal scroll bar" {
        n136 = Bundle By Name(cluster=w303, "Horizontal scroll bar"="Horizontal scroll bar") -> (w302:T12)
      }
      frame "====System====" {
      }
      frame "Panel Hidden", "Panel Insert", "Panel Show" {
        n137 = Unbundle By Name(w314) -> ("Queue List"=w313:map{string, refnum<queue>}, "Active Panel"=w310:string, "SubPanel"=w309:refnum<vi>)
        n138 = Look In Map(map=w313, key=w310) -> (value=w312:refnum<queue>)  [unwired: 1 in, 1 out]
        n139 = call "Queue In.vi"("Data"=w309, "Message"=w311, "Queue In"=w312) -> ()  [unwired: 7 in, 2 out]
      }
      frame "Show Config" {
        n140 = Unbundle By Name(w323) -> ("Queue Ref.Data Path"=w321:path)
        n141 = Build Path(base path=w321, name or relative path=path "002_DataMonitor.csv" ("名称或相对路径")) -> (appended path=w320:path)
        n142 = call <vilib>:"Check if File or Folder Exists.vi"("path"=w320) -> ("error out"=w317:errorcluster, "file or folder exists?"=w319:bool, "dup path"=w318:path)  [unwired: 8 in]
        n143 = case shown="真" w319 {
          tunnel: w318 -> [_ w327]
          tunnel: w317 -> [_ w326]
          frame False {
          }
          frame True {
            n144 = call <vilib>:"Show in File System.vi"("error in (no error)"=w326, "file or directory path"=w327) -> ()  [unwired: 9 in, 1 out]
          }
        }
      }
      frame "Panel Refresh" {
        n145 = Unbundle By Name(w330) -> ("Queue Ref.Data"=w329:refnum<queue>)
        n146 = call "Queue In.vi"("Message"="Init", "Queue In"=w329) -> ()  [unwired: 8 in, 2 out]
      }
      frame "Panel Change" {
        n147 = Unbundle By Name(w337) -> ("Vertical scroll bar"=w336:bool, "Horizontal scroll bar"=w335:bool)
        n148 = call "Queue Clear.vi"("error in (no error)"=w338, "Delete?"=TRUE, "Filter"=w339, "Queue In"=w340) -> ("error out"=w342:errorcluster, "Queue Out"=w341:refnum<queue>)  [unwired: 6 in]
        n149 = call "Refresh List Length.vi"("H"=w335, "V"=w336) -> ("error out"=w334:errorcluster)  [unwired: 8 in, 1 out]
        n150 = Or(x=w336, y=w335) -> (x .or. y?=w333:bool)
        n151 = case shown="假" w333 {
          tunnel: w334 -> [_ _]
          frame False {
            n152 = control-ref of="Main"() -> (w345:refnum<vi>)
            n153 = property class="Pane"(reference=w345, "Origin"=T13 {"Horizontal"=0, "Vertical"=0} ("原点")) -> ()  [unwired: 1 in, 2 out]
          }
          frame True {
          }
        }
      }
      frame "Send Client Refer" {
        n154 = Unbundle By Name(w349) -> ("Data"=w348:refnum<queue>)
        n155 = in-place {
          in-place-border: w350 -> [w357]
          in-place-border: [w355] -> w347
          n156 = in-place-cluster #5(w352) -> ("Queue List"=w356:map{string, refnum<queue>})
          n157 = Variant To Data(type=w356, Variant=w357) -> (data=w355:map{string, refnum<queue>})  [unwired: 1 in, 1 out]
          n158 = in-place-cluster #5("Queue List"=w355) -> (w351:T12)
        }
        n159 = call "Queue In.vi"("Data"=w347, "Message"=w346, "Queue In"=w348) -> ()  [unwired: 7 in, 2 out]
      }
      frame "Client Delete", "Client Launch" {
        n160 = Unbundle By Name(w362) -> ("Message"=w361:refnum<queue>)
        n161 = Unbundle By Name(w359) -> ("Active Panel"=w358:string)
        n162 = call "Queue In.vi"("Data"=w358, "Message"=w360, "Queue In"=w361) -> ()  [unwired: 7 in, 2 out]
      }
      frame "====User====" {
      }
      frame "All Reset", "All Set", "Digit Value Change", "Module Add", "Module Config", "Reset", "Set", "Show Edit Control" {
        n163 = Unbundle By Name(w370) -> ("ModulesRef"=w369:refnum<vi>)
        n164 = call "Modules Edit.vi"("Queue Ref"=w371, "Data"=w368, "Operate"=w372, "ModulesRef"=w369) -> ()  [unwired: 7 in, 1 out]
      }
      frame "Exit" {
        n165 = Unbundle By Name(w380) -> ("Message"=w379:refnum<queue>, "Data"=w378:refnum<queue>)
        n166 = Build Array(w379, w378) -> (w377:refnum<queue>[])
        n167 = for {
          tunnel: w377 -> [w389] mode=indexing
          tunnel: w376 -> [w388]
          n168 = call "Queue In.vi"("First"=TRUE, "Message"=w388, "Queue In"=w389) -> ()  [unwired: 7 in, 2 out]
        }
        n169 = Generate User Event(user event=w386, event data cluster=w376) -> ()  [unwired: 2 in, 2 out]
        n170 = call "Queue Clear.vi"("error in (no error)"=w382, "Queue In"=w384) -> ("error out"=w381:errorcluster, "Queue Out"=w383:refnum<queue>)  [unwired: 8 in]
      }
      frame "Quit" {
      }
    }
    n171 = call "Queue In.vi"("error in (no error)"=w269, "Message"=w268, "Queue In"=w272) -> ("error out"=w270:errorcluster, "Queue Out"=w271:refnum<queue>)  [unwired: 7 in]
  }
  n172 = call "000 Driver Message.vi"("Queue In"=w5) -> ("error out"=w22:errorcluster)  [unwired: 8 in, 2 out]
  n173 = call "Queue Release.vi"("error in (no error)"=w20, "Queue In"=w19) -> ("error out"=w23:errorcluster)  [unwired: 9 in]
  n174 = call "Queue Release.vi"("error in (no error)"=w12, "Queue In"=w11) -> ("error out"=w15:errorcluster)  [unwired: 9 in]
  n175 = Unregister For Events(event registration refnum=w8) -> (error out=w9:errorcluster)  [unwired: 1 in]
  n176 = Destroy User Event(user event=w10, error in=w9) -> (error out=w14:errorcluster)
  n177 = Call Chain() -> (call chain=w17:string[])
  n178 = Merge Errors(w14, w15, w22, w23) -> (w16:errorcluster)
  n179 = Array Size(array=w17) -> (size(s)=w18:i32)
  n180 = case shown="2.." w18 {
    tunnel: w16 -> [_ w394]
    frame 0, Default {
    }
    frame 2.. {
      n181 = invoke class="VI" method="FP.Close"(error in=w394) -> ()  [unwired: 2 in, 3 out]
    }
  }
